vi "Initialize Thread.vi"(7 "component name":string, 8 "error in (no error)":errorcluster, 10 "DSF Core.lvlibp:Thread Configuration.lvclass":refnum<class "Thread Configuration.lvclass">, 11 "UDPlog Transceiver in":refnum<class "UDPlog Transceiver.lvclass">) -> (0 "error out":errorcluster, 3 "UDPlog Transceiver out":refnum<class "UDPlog Transceiver.lvclass">)   [LabVIEW 2023, in "UDPlog.lvlib" / "UDPlog Transceiver.lvclass"]
uses:
  UDPlog Transceiver.lvclass
  Users/Public/Documents/National Instruments/NI VeriStand 2023/Custom Devices/Data Sharing Framework/Linux_x64/DSF Core.lvlibp/Classes/Configuration/Core/Thread/Thread Configuration.lvclass
  C:/Users/Public/Documents/National Instruments/NI VeriStand 2023/Custom Devices/Data Sharing Framework/Linux_x64/DSF Core.lvlibp/Classes/Configuration/Core/Core Configuration.lvclass
  Configurations/Thread/UDPlog Thread Configuration.lvclass
  Configurations/Thread/UDPlog Thread Configuration.lvclass/UDPlog Thread Configuration.ctl
  UDPlog Transceiver.lvclass/UDPlog Transceiver.ctl
  Users/Public/Documents/National Instruments/NI VeriStand 2023/Custom Devices/Data Sharing Framework/Linux_x64/DSF Core.lvlibp/Classes/Configuration/Core/Core Configuration.lvclass
  <vilib>/Utility/SystemLogging/NI_SystemLogging.lvlib
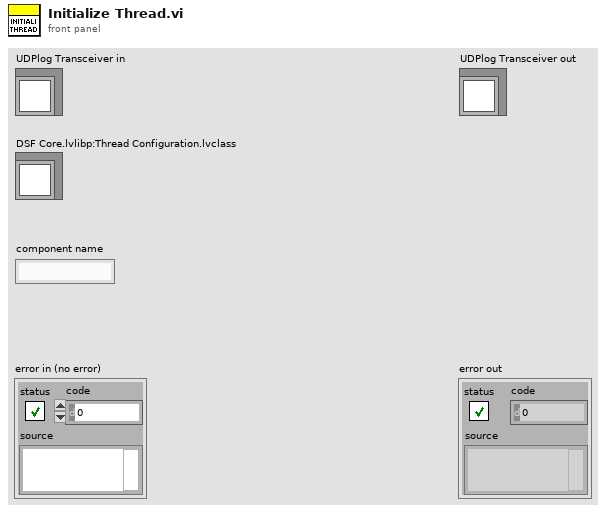
[diagram p1: front panel]
types:
  T1 = typedef "DSF Core.lvlibp/DSF Settings Info.ctl" = cluster{"component":string, "values":cluster{"key":string, "value":string}[]}
  T2 = typedef "UDPlog.lvlib/UDPlog Thread Configuration.lvclass/Thread Settings.ctl" = cluster{"local port":u16, "local address":u32}
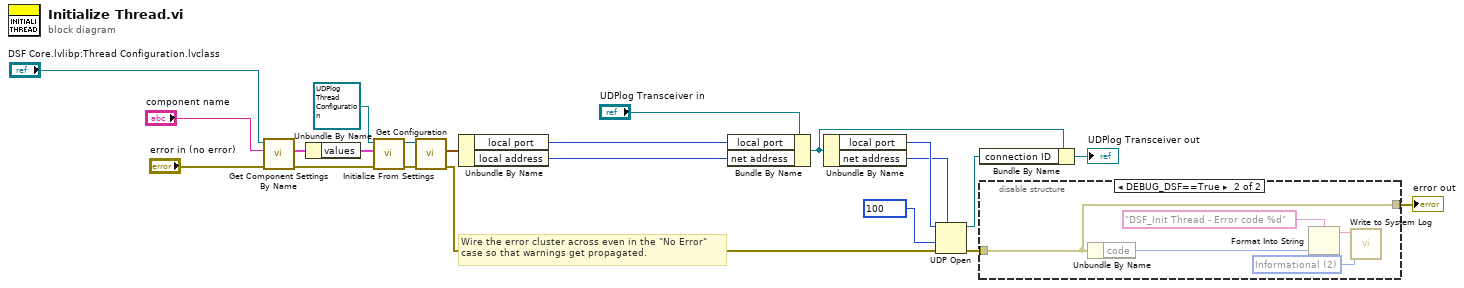
[diagram p0: block diagram]
diagram:
  # "Wire the error cluster across even in the \"No Error\"\ncase so that warnings get propagated."
  n1 = call "Get Component Settings By Name.vi"("error in (no error)"="error in (no error)", "component name"="component name", "Runtime Configuration in"="DSF Core.lvlibp:Thread Configuration.lvclass") -> ("error out"=w15:errorcluster, "component settings"=w18:T1)  [unwired: 6 in, 1 out]
  n2 = Unbundle By Name(w18) -> ("values"=w16:cluster{"key":string, "value":string}[])
  n3 = call-dynamic "Initialize From Settings.vi"("error in (no error)"=w15, "settings"=w16, "UDPlog Thread Configuration in"=refnum<class "UDPlog Thread Configuration.lvclass"> refnum) -> ("error out"=w13:errorcluster, "UDPlog Thread Configuration out"=w17:refnum<class "UDPlog Thread Configuration.lvclass">)  [unwired: 7 in]
  n4 = call "Get Configuration.vi"("error in (no error)"=w13, "UDPlog Thread Configuration in"=w17) -> ("error out"=w1:errorcluster, "thread settings"=w12:T2)  [unwired: 7 in, 1 out]
  n5 = Unbundle By Name(w12) -> ("local port"=w5:u16, "local address"=w4:u32)
  n6 = Bundle By Name(cluster="UDPlog Transceiver in", "local port"=w5, "net address"=w4) -> (w11:refnum<class "UDPlog Transceiver.lvclass">)
  n7 = Unbundle By Name(w11) -> ("local port"=w3:u16, "net address"=w2:u32)
  n8 = UDP Open(7:w2, 8:w1, 9:100 ("timeout ms (25000)"), 11:w3) -> (port=w6:refnum<k16>, 0:w9:errorcluster)  [unwired: 1 in, 1 out]
  n9 = Bundle By Name(cluster=w11, "connection ID"=w6) -> (→"UDPlog Transceiver out":refnum<class "UDPlog Transceiver.lvclass">)
  n10 = disable-structure shown="DEBUG_DSF==True" {
    disable-tunnel: w9 -> [_ w25]
    disable-tunnel: [_ w25] -> w8
    frame condition #0 (active) {
    }
    frame condition #1 {
      w23 = 2 items=["Error", "Warning", "Informational"] ("severity")
      n11 = Unbundle By Name(w25) -> ("code"=w24:i32)
      n12 = Format Into String(format string="DSF_Init Thread - Error code %d", w24) -> (resulting string=w26:string)  [unwired: 2 in, 1 out]
      n13 = call <vilib>:"Write to System Log.vi"("severity"=w23, "message"=w26) -> ()  [unwired: 9 in, 1 out]
    }
  }
  "error out" <- w8
